vi "Log.vi"(7 "severity":i32(ring)=2 caption="severity (Error)" items=["Error", "Warning", "Info"], 8 "error in (no error)":errorcluster, 9 "Data":variant, 11 "Module in":refnum<class "Module.lvclass">) -> (0 "error out":errorcluster, 3 "Module out":refnum<class "Module.lvclass">)   [LabVIEW 2020, in "Module.lvclass"]
uses:
  Module.lvclass
  Module.lvclass/Module.ctl
  Logging/Logging.lvclass
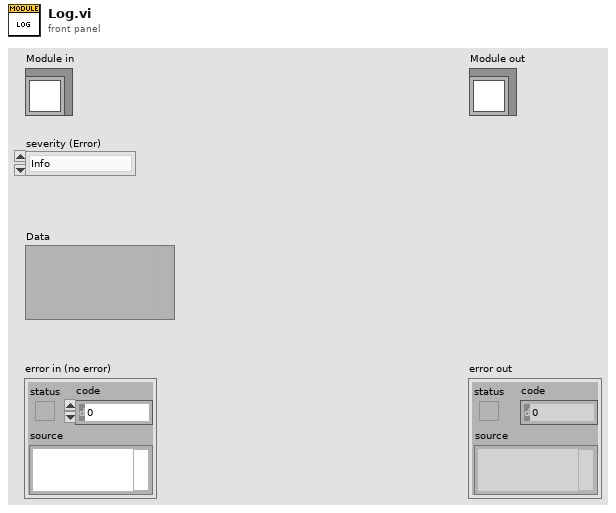
[diagram p1: front panel]
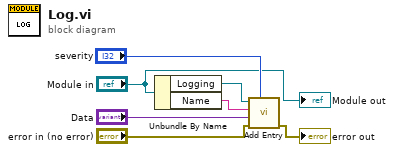
[diagram p0: block diagram]
diagram:
  n1 = Unbundle By Name("Module in") -> ("Logging"=w3:refnum<class "Logging.lvclass">, "Name"=w1:string)
  n2 = call "Add Entry.vi"("severity"="severity", "error in (no error)"="error in (no error)", "Data"="Data", "Origin"=w1, "Logging in"=w3) -> ("error out"=→"error out":errorcluster)  [unwired: 5 in, 1 out]
  "Module out" <- "Module in"
